vi "Configure Channel Vertical.vi"(7 "Offset (0)":dbl, 8 "error in (no error)":errorcluster, 9 "Scale (1)":dbl=1.0, 10 "Channel (1: Channel 1)":i32(ring)=1 items=["Channel 1"=1, "Channel 2"=2, "Channel 3"=3, "Channel 4"=4], 11 "VISA resource name":refnum<visa-resource-name>) -> (0 "error out":errorcluster, 3 "VISA resource name out":refnum<visa-resource-name>)   [LabVIEW 2015]
doc: "Configures the vertical setting for channel."
uses:
  ZhiYuan ZDS Series for TCP.lvlib
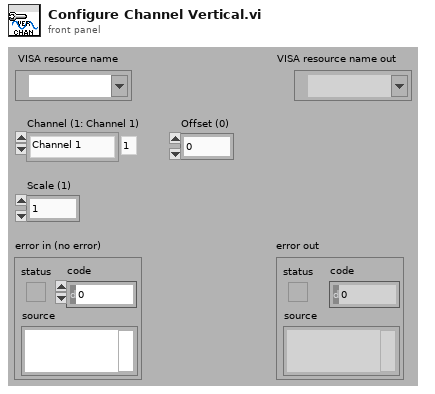
[diagram p1: front panel]
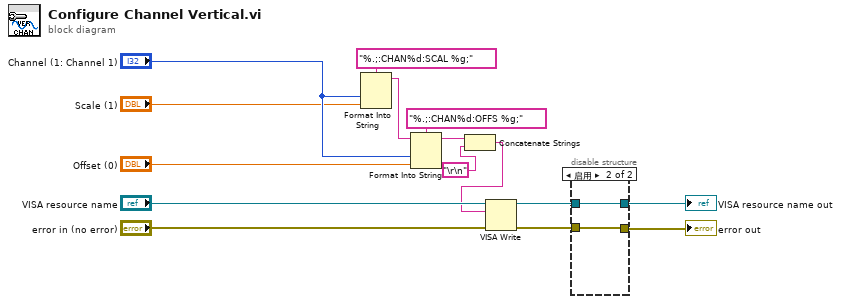
[diagram p0: block diagram]
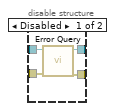
[diagram p2: hidden frame]
diagram:
  n1 = Format Into String(format string="%.;:CHAN%d:SCAL %g;", "Channel (1: Channel 1)", "Scale (1)") -> (resulting string=w12:string)  [unwired: 2 in, 1 out]
  n2 = Format Into String(format string="%.;:CHAN%d:OFFS %g;", initial string=w12, "Channel (1: Channel 1)", "Offset (0)") -> (resulting string=w3:string)  [unwired: 1 in, 1 out]
  n3 = Concatenate Strings(w3, "\r\n") -> (w1:string)
  n4 = VISA Write(VISA resource name="VISA resource name", write buffer=w1, error in (no error)="error in (no error)") -> (VISA resource name out=w7:refnum<visa-resource-name>, error out=w6:errorcluster)  [unwired: 1 out]
  n5 = disable-structure shown="启用" {
    disable-tunnel: w7 -> [w19 w21]
    disable-tunnel: w6 -> [w18 w20]
    disable-tunnel: [w17 w21] -> w5
    disable-tunnel: [w16 w20] -> w4
    frame Disabled {
      n6 = call "Error Query.vi"("error in (no error)"=w18, "VISA resource name"=w19) -> ("error out"=w16:errorcluster, "VISA resource name out"=w17:refnum<visa-resource-name>)  [unwired: 6 in, 2 out]
    }
    frame Enabled {
    }
  }
  "VISA resource name out" <- w5
  "error out" <- w4
